vi "Recall Bar Sample Hall Voltages.vi"() -> (2 "Bar Sample Hall Voltage":dbl[](array[numeric]))   [LabVIEW 2016, in "Hall Effect Library.lvlib"]
uses:
  Hall Effect Library.lvlib
  Private/Global Variables/Hall Effect Data.vi
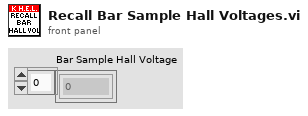
[diagram p1: front panel]
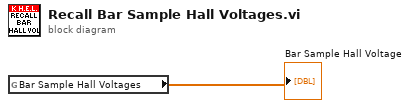
[diagram p0: block diagram]
diagram:
  n1 = global read "Hall Effect Data.vi" "Bar Sample Hall Voltages"() -> (→"Bar Sample Hall Voltage":dbl[])
